vi "Get Image Data Size.vi"(9 "Depth":i32, 10 "Height":i32, 11 "Width":i32) -> (3 "Image Data Size":i32)   [LabVIEW 2020, in "G-Image.lvlib"]
uses:
  G-Image.lvlib
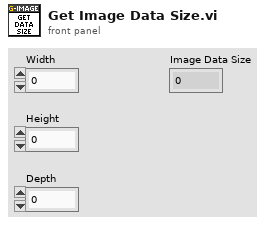
[diagram p1: front panel]
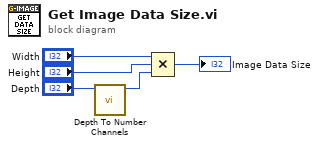
[diagram p0: block diagram]
diagram:
  n1 = call "Depth To Number Channels.vi"("Depth"="Depth") -> ("Channels"=w2:i32)  [unwired: 10 in]
  n2 = Compound Arithmetic op=MULTIPLY("Width", "Height", w2) -> (→"Image Data Size":i32)
